vi "Save Angle (SubVI).vi"(1 "Angle":fxp<+/-,16,3> format="%.14g", 2 "In Valid?":bool, 3 "Done?":bool) -> ()   [LabVIEW 2015]
uses:
  <vilib>/rvi/Memory/Memory_Emulation/nirvimemoryFastEmulation.vi
  <vilib>/rvi/Memory/Memory_Emulation/nirvimemoryEmulation.vi
  <vilib>/rvi/Emulation/niFpgaEmulationIsFPGAContextNoSignature.vi
  <vilib>/rvi/DataTransferAndStorage/Container/Common/niFpgaContainerGetUniqueNameForEmu.vi
  <vilib>/rvi/Emulation/niFpgaProcessEmulError.vi
  <vilib>/rvi/Emulation/niFpgaSctlEmulationGetInTimedLoop.vi
  <vilib>/rvi/errors/nirviReportUnexpectedCaseInternalError (U32).vi
  <vilib>/rvi/DataTransferAndStorage/Container/XNode/niFpgaContainer.xnode
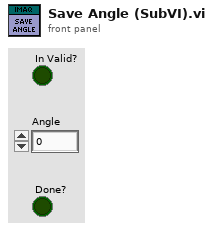
[diagram p1: front panel]
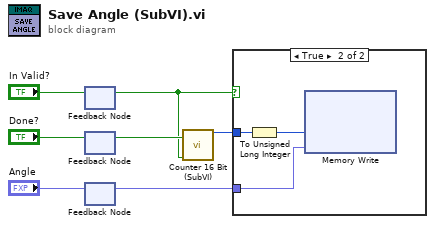
[diagram p0: block diagram]
diagram:
  n1 = feedback-in #1("In Valid?") -> ()
  n2 = feedback #1() -> (w2:bool)  [unwired: 1 in]
  n3 = feedback-in #2("Done?") -> ()
  n4 = feedback #2() -> (w3:bool)  [unwired: 1 in]
  n5 = feedback-in #3("Angle") -> ()
  n6 = feedback #3() -> (w1:fxp<+/-,16,3>)  [unwired: 1 in]
  n7 = call "Counter 16 Bit (SubVI).vi"("RESET"=w3, "Enable"=w2) -> ("Count"=w4:u16)  [unwired: 11 in, 2 out]
  n8 = case shown="True" w2 {
    tunnel: w1 -> [_ w8]
    tunnel: w4 -> [_ w10]
    frame False {
    }
    frame True {
      n9 = To Unsigned Long Integer(number=w10) -> (unsigned 32bit integer=w9:u32)
      n10 = xnode ("Memory Write")("Address"=w9, "Data"=w8) -> ()  [unwired: 1 in, 1 out]
    }
  }
